vi "Channel 1  Adc Conversion.vi"(8 "Error In":errorcluster, 11 "Adc Convertor In":refnum<class "Adc Convertor.lvclass">) -> (0 "Error Out":errorcluster, 3 "Adc Convertor Out":refnum<class "Adc Convertor.lvclass">)   [LabVIEW 2021, in "Adc Convertor.lvclass"]
doc: "This VI converts the analog data to digital data of channel 1."
uses:
  Adc Convertor.lvclass
  <vilib>/numeric/Random Number (Range) DBL.vi
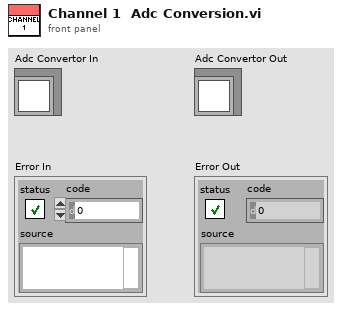
[diagram p1: front panel]
types:
  T1 = typedef "Channel Data.ctl" = cluster{"Channel 1 U8  Array":u8[], "Channel 2 U8  Array ":u8[], "Channel 3 U8  Array":u8[], "Channel 4 U8  Array":u8[]}
  T2 = typedef "ADC Type.ctl" = cluster{"Channels":string, "Range":dbl, "Resolution":dbl, "Sampling Rate":dbl}
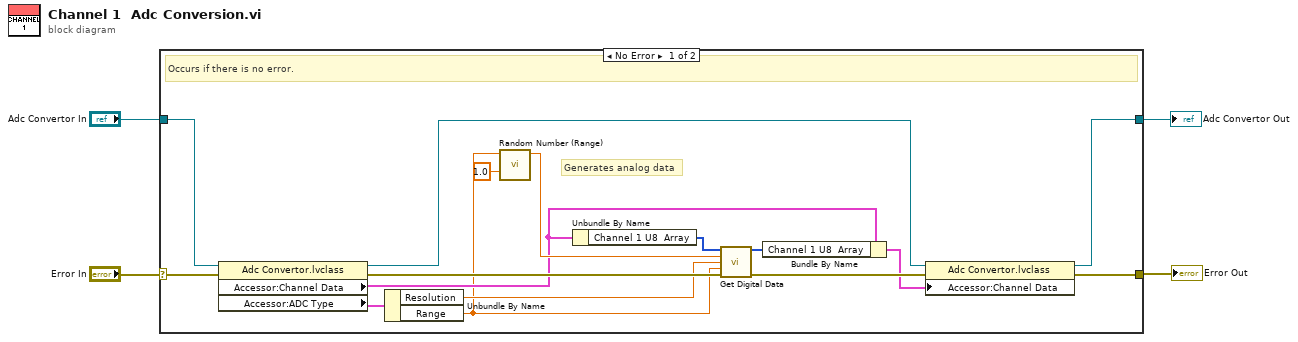
[diagram p0: block diagram]
diagram:
  n1 = case shown="No Error" "Error In" {
    selector: "Error In" -> [w12 w22]
    tunnel: [w11 w22] -> w3
    tunnel: [w9 w21] -> w1
    tunnel: "Adc Convertor In" -> [w10 w21]
    frame No Error {
      # "Generates analog data"
      # "Occurs if there is no error."
      n2 = property class="Adc Convertor.lvclass"(reference=w10, error in=w12) -> (reference out=w7:refnum<class "Adc Convertor.lvclass">, error out=w19:errorcluster, "Accessor:Channel Data"=w6:T1, "Accessor:ADC Type"=w17:T2)
      n3 = Unbundle By Name(w17) -> ("Resolution"=w16:dbl, "Range"=w5:dbl)
      n4 = call-poly <vilib>:"Random Number (Range).vi"("lower bound (0)"=1.0, "upper bound (100)"=w5) -> ("number"=w13:dbl)  [unwired: 9 in]
      n5 = Unbundle By Name(w6) -> ("Channel 1 U8  Array"=w18:u8[])
      n6 = call "Get Digital Data.vi"("Input Array"=w18, "Analog Input"=w13, "Resolution"=w16, "Range"=w5, "Error In"=w19) -> ("Output Array"=w8:u8[], "Error Out"=w20:errorcluster)  [unwired: 9 in]
      n7 = Bundle By Name(cluster=w6, "Channel 1 U8  Array"=w8) -> (w15:T1)
      n8 = property class="Adc Convertor.lvclass"(reference=w7, error in=w20, "Accessor:Channel Data"=w15) -> (reference out=w9:refnum<class "Adc Convertor.lvclass">, error out=w11:errorcluster)
    }
    frame Error {
      # "Occurs if there is any error."
    }
  }
  "Error Out" <- w3
  "Adc Convertor Out" <- w1
